vi "Log Variant Data to File.vi"(8 "error in (no error)":errorcluster, 10 "UUID":string, 11 "CubeLogger in":refnum<class "CubeLogger.lvclass">) -> (0 "error out":errorcluster, 2 "Finished?":bool, 3 "CubeLogger out":refnum<class "CubeLogger.lvclass">)   [LabVIEW 2018, in "CubeLogger.lvclass"]
uses:
  CubeLogger.lvclass
  CubeLogger.lvclass/CubeLogger.ctl
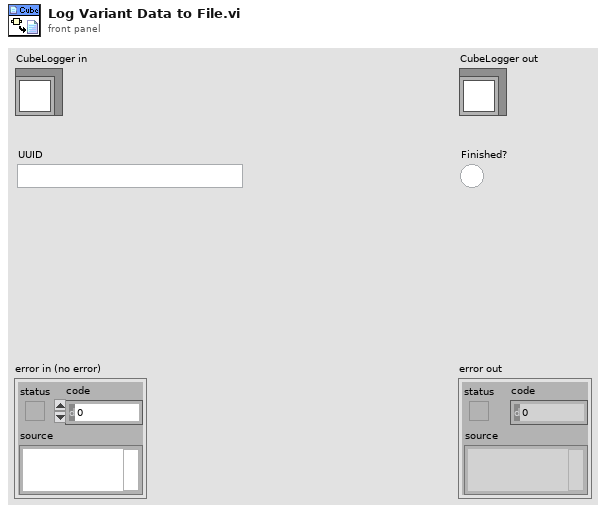
[diagram p1: front panel]
types:
  T1 = typedef "CubeLogger.lvclass/Endianness.ctl" = enum16{"big-endian, network order", "native, host order", "little-endian"}
  T2 = typedef "CubeLogger.lvclass/Dataset.ctl" = cluster{"name":string, "path":string, "size":i32[], "type":enum16{"single", "double", "uint8", "uint16", "uint32", "uint64", "int8", "int16", "int32", "int64"}, "mfmt":string}
  T3 = typedef "NI_Data Type.lvlib/Data Type.ctl" = enum8{"Invalid Type", "Void", "I8", "I16", "I32", "I64", "U8", "U16", "U32", "U64", "Single Float", "Double Float", "Extended Float", "Single Complex", "Double Complex", "Extended Complex", "Enum U8", "Enum U16", "Enum U32", "Enum U64", "Single Float With Unit", "Double Float With Unit", "Extended Float With Unit", "Single Complex with Unit", "Double Complex with Unit", "Extended Complex with Unit", "Boolean", "String", "Path", "Picture", "Tag", "Array", "Cluster", "Variant", "LV Variant", "Waveform", "Timestamp", "Digital Waveform", "Digital Data", "ExpressData", "Refnum", "External Data", "VI", "Poly VI", "LabVIEW Class Instance", "Fixed Point"}
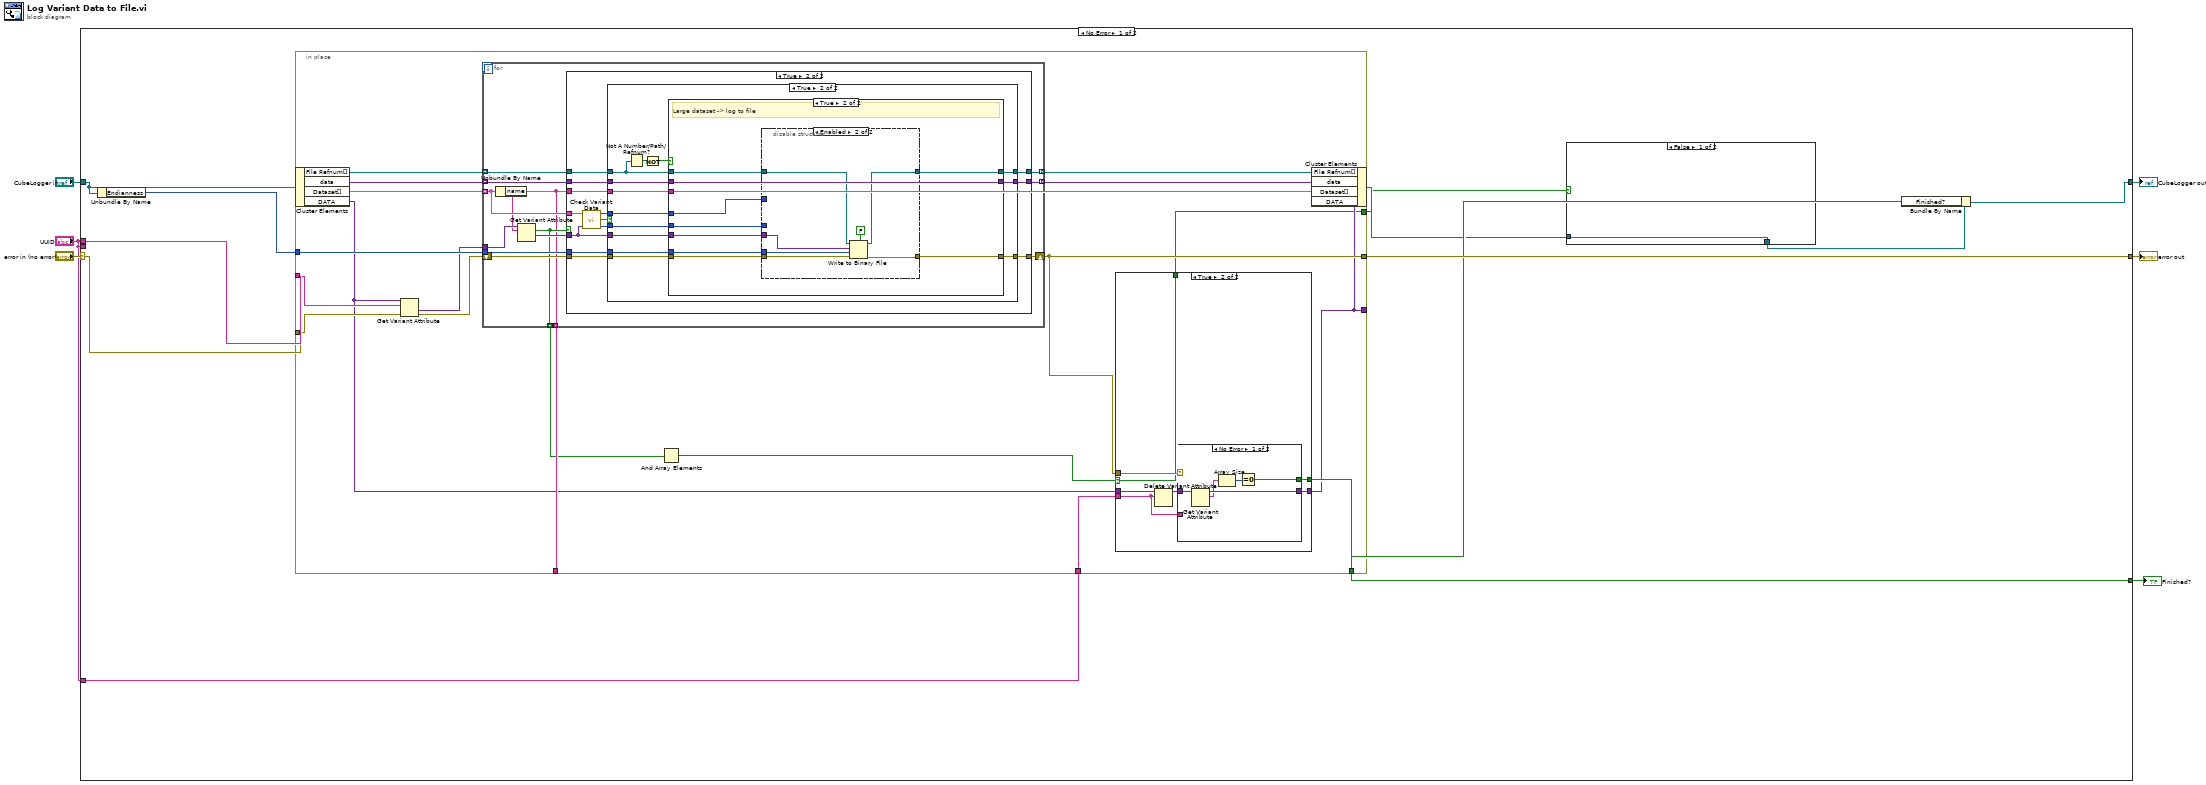
[diagram p0: block diagram]
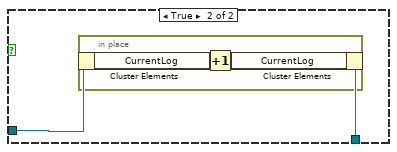
[diagram p2: hidden frame]
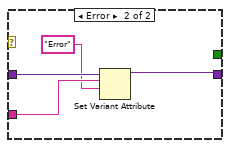
[diagram p4: hidden frame]
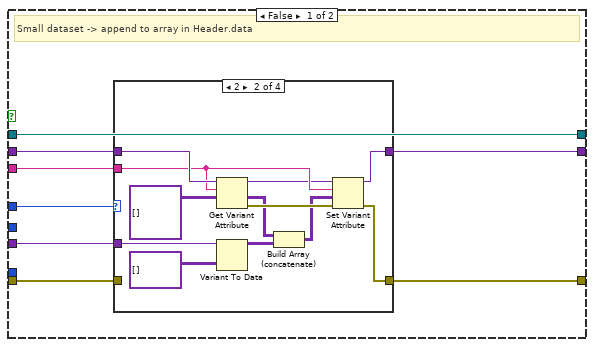
[diagram p7: hidden frame]
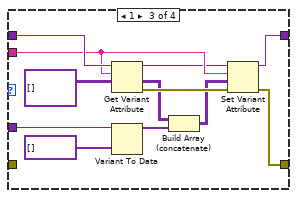
[diagram p9: hidden frame]
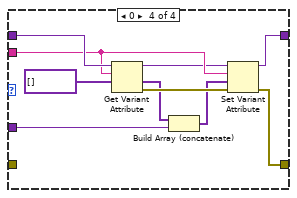
[diagram p10: hidden frame]
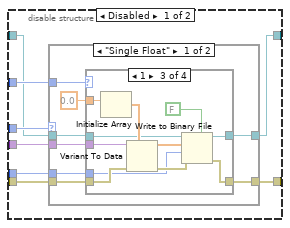
[diagram p11: hidden frame]
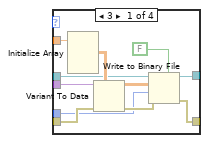
[diagram p12: hidden frame]
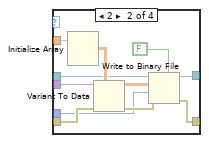
[diagram p13: hidden frame]
diagram:
  n1 = case shown="No Error" "error in (no error)" {
    selector: "error in (no error)" -> [w12 w217]
    tunnel: [w15 w217] -> w3
    tunnel: [w14 w218] -> w4
    tunnel: "CubeLogger in" -> [w17 w218]
    tunnel: "UUID" -> [_ _]
    tunnel: [w10 _] -> w2
    tunnel: "UUID" -> [w13 _]
    tunnel: "UUID" -> [w11 _]
    frame No Error {
      n2 = Unbundle By Name(w17) -> ("Endianness"=w16:T1)
      n3 = in-place {
        in-place-border: w16 -> [w37]
        in-place-border: [w36] -> w15
        in-place-border: [w34] -> _
        in-place-border: w13 -> [w33]
        in-place-border: w12 -> [w32]
        in-place-border: w11 -> [w28]
        in-place-border: [w27] -> w10
        in-place-border: [w26] -> _
        in-place-border: [w25] -> w7
        n4 = in-place-cluster #1(w17) -> ("File Refnum[]"=w40:refnum<file>[], "data"=w39:variant[], "Dataset[]"=w35:T2[], "DATA"=w29:variant)
        n5 = Get Variant Attribute(Variant=w29, name=w33, error in=w32) -> (value=w31:variant, error out=w30:errorcluster)  [unwired: 1 in, 2 out]
        n6 = for {
          tunnel: [w71] -> w41 mode=indexing
          tunnel: w40 -> [w68] mode=indexing
          tunnel: w39 -> [w67] mode=indexing
          tunnel: w31 -> [w63]
          tunnel: [w70] -> w38 mode=indexing
          tunnel: w35 -> [w64] mode=indexing
          tunnel: w37 -> [w66]
          shift-right: [w65] -> w36
          shift-left: w30 -> [w69]
          tunnel: [w61] -> w24 mode=indexing
          tunnel: [w60] -> w34 mode=indexing
          n7 = Unbundle By Name(w64) -> ("name"=w60:string)
          n8 = Get Variant Attribute(Variant=w63, name=w60) -> (found=w61:bool, value=w62:variant)  [unwired: 2 in, 2 out]
          n9 = case shown="True" w61 {
            tunnel: [w73 w87] -> w71
            tunnel: [w72 w86] -> w70
            tunnel: w69 -> [w74 w85]
            tunnel: w68 -> [w73 w84]
            tunnel: w67 -> [w72 w83]
            tunnel: w66 -> [_ w82]
            tunnel: [w74 w81] -> w65
            tunnel: w64 -> [_ w79]
            tunnel: w60 -> [_ w78]
            tunnel: w62 -> [_ w77]
            frame False {
            }
            frame True {
              n10 = call "Check Variant Data.vi"("Variant Data"=w77, "Dataset"=w79) -> ("Element Type"=w75:T3, "Valid Type?"=w80:bool, "Number of Dimensions"=w76:i32)  [unwired: 1 in]
              n11 = case shown="True" w80 {
                tunnel: [w90 w103] -> w87
                tunnel: [w89 w102] -> w86
                tunnel: w85 -> [w88 w101]
                tunnel: w84 -> [w90 w99]
                tunnel: w83 -> [w89 w97]
                tunnel: w82 -> [_ w96]
                tunnel: [w88 w95] -> w81
                tunnel: w78 -> [_ w94]
                tunnel: w77 -> [_ w93]
                tunnel: w76 -> [_ w92]
                tunnel: w75 -> [_ w91]
                frame False {
                  # "RAISE ERROR HERE"
                }
                frame True {
                  n12 = Not A Number/Path/Refnum?(number/path/refnum=w99) -> (NaN/Path/Refnum?=w100:bool)
                  n13 = Not(x=w100) -> (.not. x?=w98:bool)
                  n14 = case shown="True" w98 {
                    tunnel: [w111 w148] -> w103
                    tunnel: w99 -> [w111 w149]
                    tunnel: [w108 w152] -> w102
                    tunnel: w101 -> [w107 w150]
                    tunnel: w94 -> [w109 _]
                    tunnel: w97 -> [w110 w152]
                    tunnel: w96 -> [_ w153]
                    tunnel: [w106 w151] -> w95
                    tunnel: w93 -> [w105 w154]
                    tunnel: w92 -> [w104 w156]
                    tunnel: w91 -> [_ w155]
                    frame False {
                      # "Small dataset -> append to array in Header.data"
                      n15 = case shown="2" w104 {
                        tunnel: w110 -> [w113 w125 w137 w147]
                        tunnel: w109 -> [_ w124 w136 w146]
                        tunnel: [w113 w122 w134 w144] -> w108
                        tunnel: w107 -> [w112 _ _ _]
                        tunnel: [w112 w119 w131 w141] -> w106
                        tunnel: w105 -> [_ w115 w127 w138]
                        frame Default {
                          # "RAISE ERROR"
                        }
                        frame 2 {
                          n16 = Get Variant Attribute(Variant=w125, name=w124, default value (empty Variant)=variant[][][] []) -> (duplicate Variant=w123:variant, value=w118:variant[][][], error out=w120:errorcluster)  [unwired: 1 in, 1 out]
                          n17 = Variant To Data(type=variant[][] [], Variant=w115) -> (data=w116:variant[][])  [unwired: 1 in, 1 out]
                          n18 = Build Array (concatenate)(w118, w116) -> (w117:variant[][][])
                          n19 = Set Variant Attribute(Variant=w123, name=w124, value=w117, error in=w120) -> (Variant out=w122:variant, error out=w119:errorcluster)  [unwired: 1 out]
                        }
                        frame 1 {
                          n20 = Get Variant Attribute(Variant=w137, name=w136, default value (empty Variant)=variant[][] []) -> (duplicate Variant=w135:variant, value=w130:variant[][], error out=w132:errorcluster)  [unwired: 1 in, 1 out]
                          n21 = Variant To Data(type=variant[] [], Variant=w127) -> (data=w128:variant[])  [unwired: 1 in, 1 out]
                          n22 = Build Array (concatenate)(w130, w128) -> (w129:variant[][])
                          n23 = Set Variant Attribute(Variant=w135, name=w136, value=w129, error in=w132) -> (Variant out=w134:variant, error out=w131:errorcluster)  [unwired: 1 out]
                        }
                        frame 0 {
                          n24 = Get Variant Attribute(Variant=w147, name=w146, default value (empty Variant)=variant[] []) -> (duplicate Variant=w145:variant, value=w140:variant[], error out=w142:errorcluster)  [unwired: 1 in, 1 out]
                          n25 = Build Array (concatenate)(w140, w138) -> (w139:variant[])
                          n26 = Set Variant Attribute(Variant=w145, name=w146, value=w139, error in=w142) -> (Variant out=w144:variant, error out=w141:errorcluster)  [unwired: 1 out]
                        }
                      }
                    }
                    frame True {
                      # "Large dataset -> log to file"
                      n27 = disable-structure shown="Enabled" {
                        disable-tunnel: w156 -> [w164 _]
                        disable-tunnel: w155 -> [w163 _]
                        disable-tunnel: w154 -> [w162 w211]
                        disable-tunnel: w153 -> [w161 w210]
                        disable-tunnel: [w160 w215] -> w151
                        disable-tunnel: w150 -> [w159 w216]
                        disable-tunnel: w149 -> [w158 w214]
                        disable-tunnel: [w157 w213] -> w148
                        frame Disabled {
                          n28 = case shown="\"Single Float\"" w163 {
                            tunnel: w164 -> [w172 _]
                            tunnel: w162 -> [w170 _]
                            tunnel: w159 -> [w169 w209]
                            tunnel: [w168 w209] -> w160
                            tunnel: w161 -> [w167 _]
                            tunnel: [w166 w208] -> w157
                            tunnel: w158 -> [w165 w208]
                            frame "Single Float" {
                              n29 = case shown="1" w172 {
                                tunnel: sgl 0.0 -> [w182 w193 w204 _]
                                tunnel: w170 -> [w181 w192 w203 _]
                                tunnel: w169 -> [w179 w190 w201 w206]
                                tunnel: [w178 w189 w200 w206] -> w168
                                tunnel: w167 -> [w177 w188 w199 _]
                                tunnel: w165 -> [w176 w187 w198 w207]
                                tunnel: [w175 w186 w197 w207] -> w166
                                frame 3 {
                                n30 = Initialize Array(w182) -> (w183:sgl[][][])  [unwired: 3 in]
                                n31 = Variant To Data(error in=w179, type=w183, Variant=w181) -> (data=w174:sgl[][][], error out=w180:errorcluster)
                                n32 = Write to Binary File(file (use dialog)=w176, data=w174, error in=w180, 5:FALSE ("prepend array or string size? (T)"), 9:w177) -> (refnum out=w175:refnum<file>, error out=w178:errorcluster)  [unwired: 1 in, 1 out]
                                }
                                frame 2 {
                                n33 = Initialize Array(w193) -> (w194:sgl[][])  [unwired: 2 in]
                                n34 = Variant To Data(error in=w190, type=w194, Variant=w192) -> (data=w185:sgl[][], error out=w191:errorcluster)
                                n35 = Write to Binary File(file (use dialog)=w187, data=w185, error in=w191, 5:FALSE ("prepend array or string size? (T)"), 9:w188) -> (refnum out=w186:refnum<file>, error out=w189:errorcluster)  [unwired: 1 in, 1 out]
                                }
                                frame 1 {
                                n36 = Initialize Array(w204) -> (w205:sgl[])  [unwired: 1 in]
                                n37 = Variant To Data(error in=w201, type=w205, Variant=w203) -> (data=w196:sgl[], error out=w202:errorcluster)
                                n38 = Write to Binary File(file (use dialog)=w198, data=w196, error in=w202, 5:FALSE ("prepend array or string size? (T)"), 9:w199) -> (refnum out=w197:refnum<file>, error out=w200:errorcluster)  [unwired: 1 in, 1 out]
                                }
                                frame Default {
                                }
                              }
                            }
                            frame Default {
                            }
                          }
                        }
                        frame Enabled {
                          n39 = Write to Binary File(file (use dialog)=w214, data=w211, error in=w216, 5:FALSE ("prepend array or string size? (T)"), 9:w210) -> (refnum out=w213:refnum<file>, error out=w215:errorcluster)  [unwired: 1 in, 1 out]
                        }
                      }
                    }
                  }
                }
              }
            }
          }
        }
        n40 = And Array Elements(Boolean array=w24) -> (logical AND=w23:bool)
        n41 = case shown="True" w23 {
          selector: w23 -> [w42 w44]
          tunnel: w36 -> [_ w50]
          tunnel: w29 -> [w43 w49]
          tunnel: [w43 w47] -> w26
          tunnel: w28 -> [_ w46]
          tunnel: [_ w45] -> w27
          tunnel: [w42 w44] -> w25
          frame False {
          }
          frame True {
            n42 = Delete Variant Attribute(6:w46, 7:w49) -> (3:w48:variant)  [unwired: 1 in, 2 out]
            n43 = case shown="No Error" w50 {
              tunnel: w48 -> [w55 w58]
              tunnel: [w54 w59] -> w47
              tunnel: w46 -> [_ w57]
              tunnel: [w51 _] -> w45
              frame No Error {
                n44 = Get Variant Attribute(Variant=w55) -> (duplicate Variant=w54:variant, names=w53:string[])  [unwired: 3 in, 2 out]
                n45 = Array Size(array=w53) -> (size(s)=w52:i32)
                n46 = Equal To 0?(x=w52) -> (x = 0?=w51:bool)
              }
              frame Error {
                n47 = Set Variant Attribute(Variant=w58, name=w57, value="Error") -> (Variant out=w59:variant)  [unwired: 1 in, 2 out]
              }
            }
          }
        }
        n48 = in-place-cluster #1("File Refnum[]"=w41, "data"=w38, "Dataset[]"=w35, "DATA"=w26) -> (w8:refnum<class "CubeLogger.lvclass">)
      }
      n49 = case shown="False" w7 {
        tunnel: w8 -> [w18 w20]
        tunnel: [w18 w19] -> w9
        frame False {
        }
        frame True {
          n50 = in-place {
            n51 = in-place-cluster #2(w20) -> ("CurrentLog"=w22:i32)
            n52 = Increment(x=w22) -> (x+1=w21:i32)
            n53 = in-place-cluster #2("CurrentLog"=w21) -> (w19:refnum<class "CubeLogger.lvclass">)
          }
        }
      }
      n54 = Bundle By Name(cluster=w9, "Finished?"=w10) -> (w14:refnum<class "CubeLogger.lvclass">)
    }
    frame Error {
    }
  }
  "error out" <- w3
  "CubeLogger out" <- w4
  "Finished?" <- w2
